vi "Helium Fridge Cool-Down.vi"() -> ()   [LabVIEW 2014]
uses:
  <vilib>/express/express shared/transition.llb/Dynamic To Waveform Array.vi
  <vilib>/express/express signal manip/GetorSetDDTAttributes/Set DDT Attributes/SetT0.vi
  <vilib>/express/express shared/transition.llb/Waveform Array To Dynamic.vi
  <vilib>/express/express signal manip/GetorSetDDTAttributes/Set DDT Attributes/Set DDT Properties.xnode
panel:
  out "Lab Time":string
  out "Most Recent Error":string
  out "Last Sweep Start Time":string
  out "Most Recent Error":string
  out "Last Measurement Taken":string
  out "Run Start Time":string
  in  "Seconds Between\nMeasurements":dbl=30.0
  out "All Clear":bool=TRUE
  out "Error":bool
  out "Heartbeat":bool
  out "?":bool
  in  "stop":bool
  out "Input Triangle Wave":dynamicdata(graph)
  out "Modulator":dynamicdata(graph)
  out "Q Meter":cluster{"Y":dbl[], "Y":dbl[]}[](graph)
  in  "# of Sweeps":dbl=100.0
  out "Resistance Strip Chart":dynamicdata(graph)
  out "Temperature Strip Chart":dynamicdata(graph)
  in  "Heartbeat":bool
  in  "Temp Strip Chart":bool
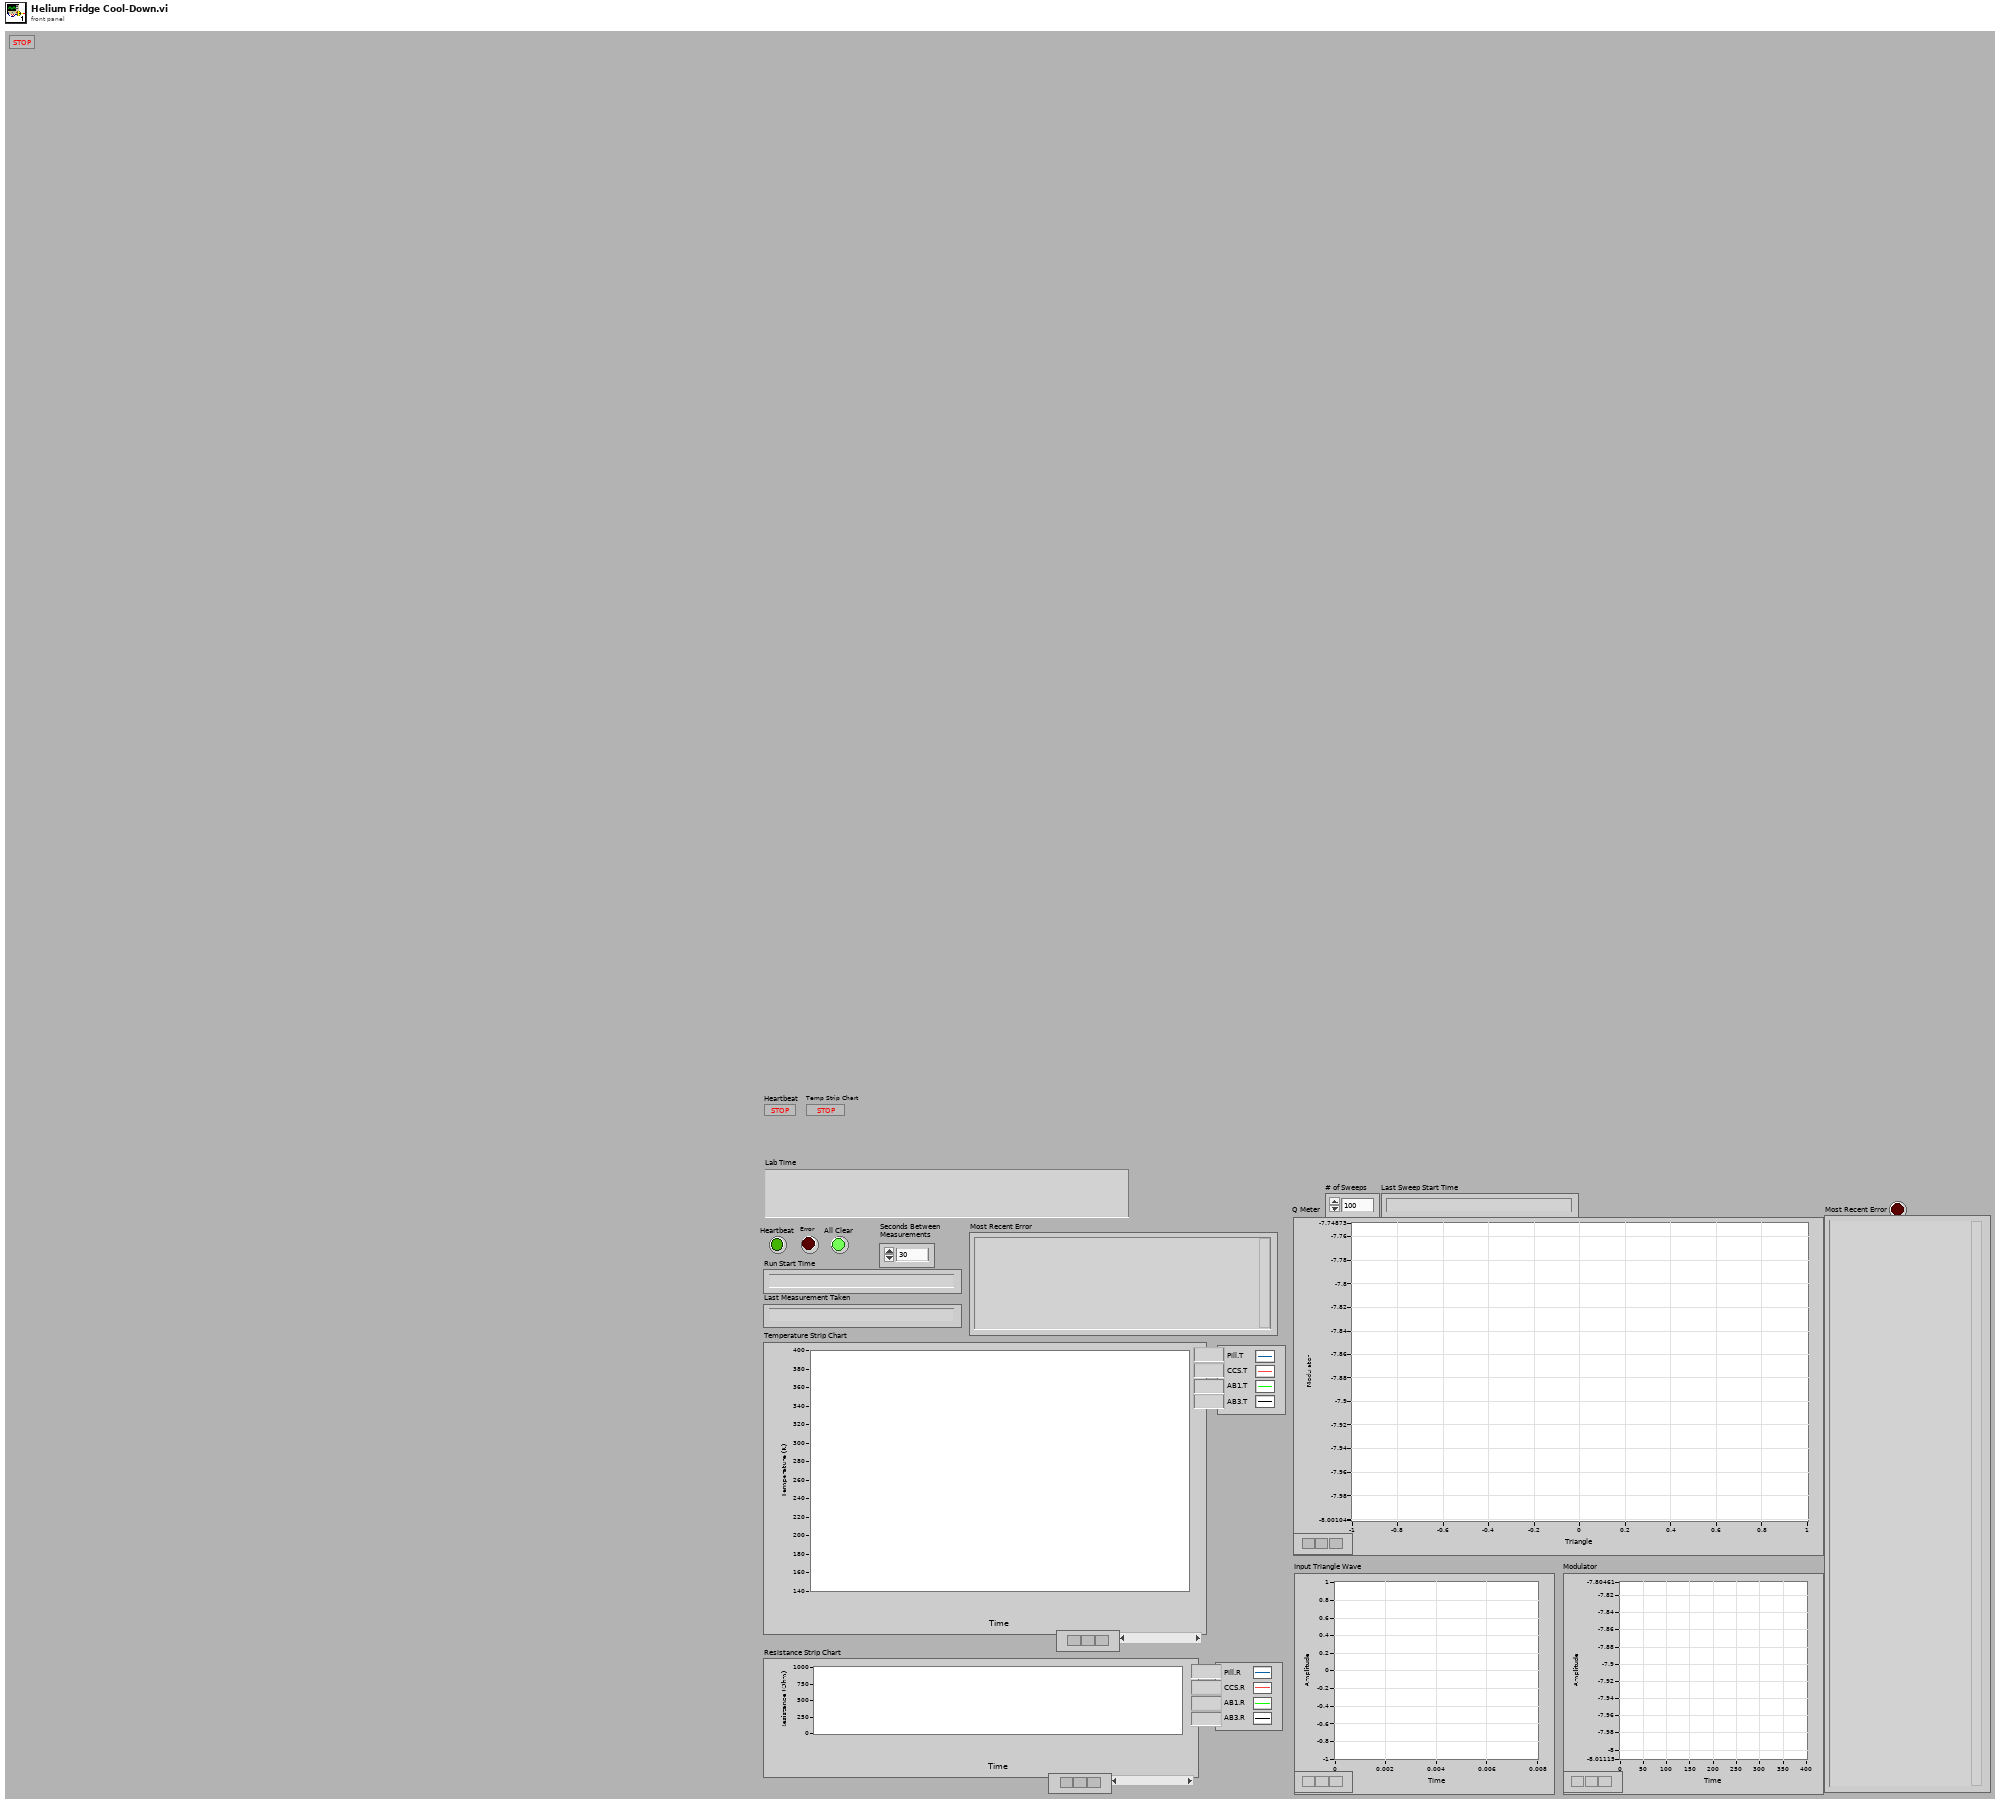
[diagram p1: front panel]
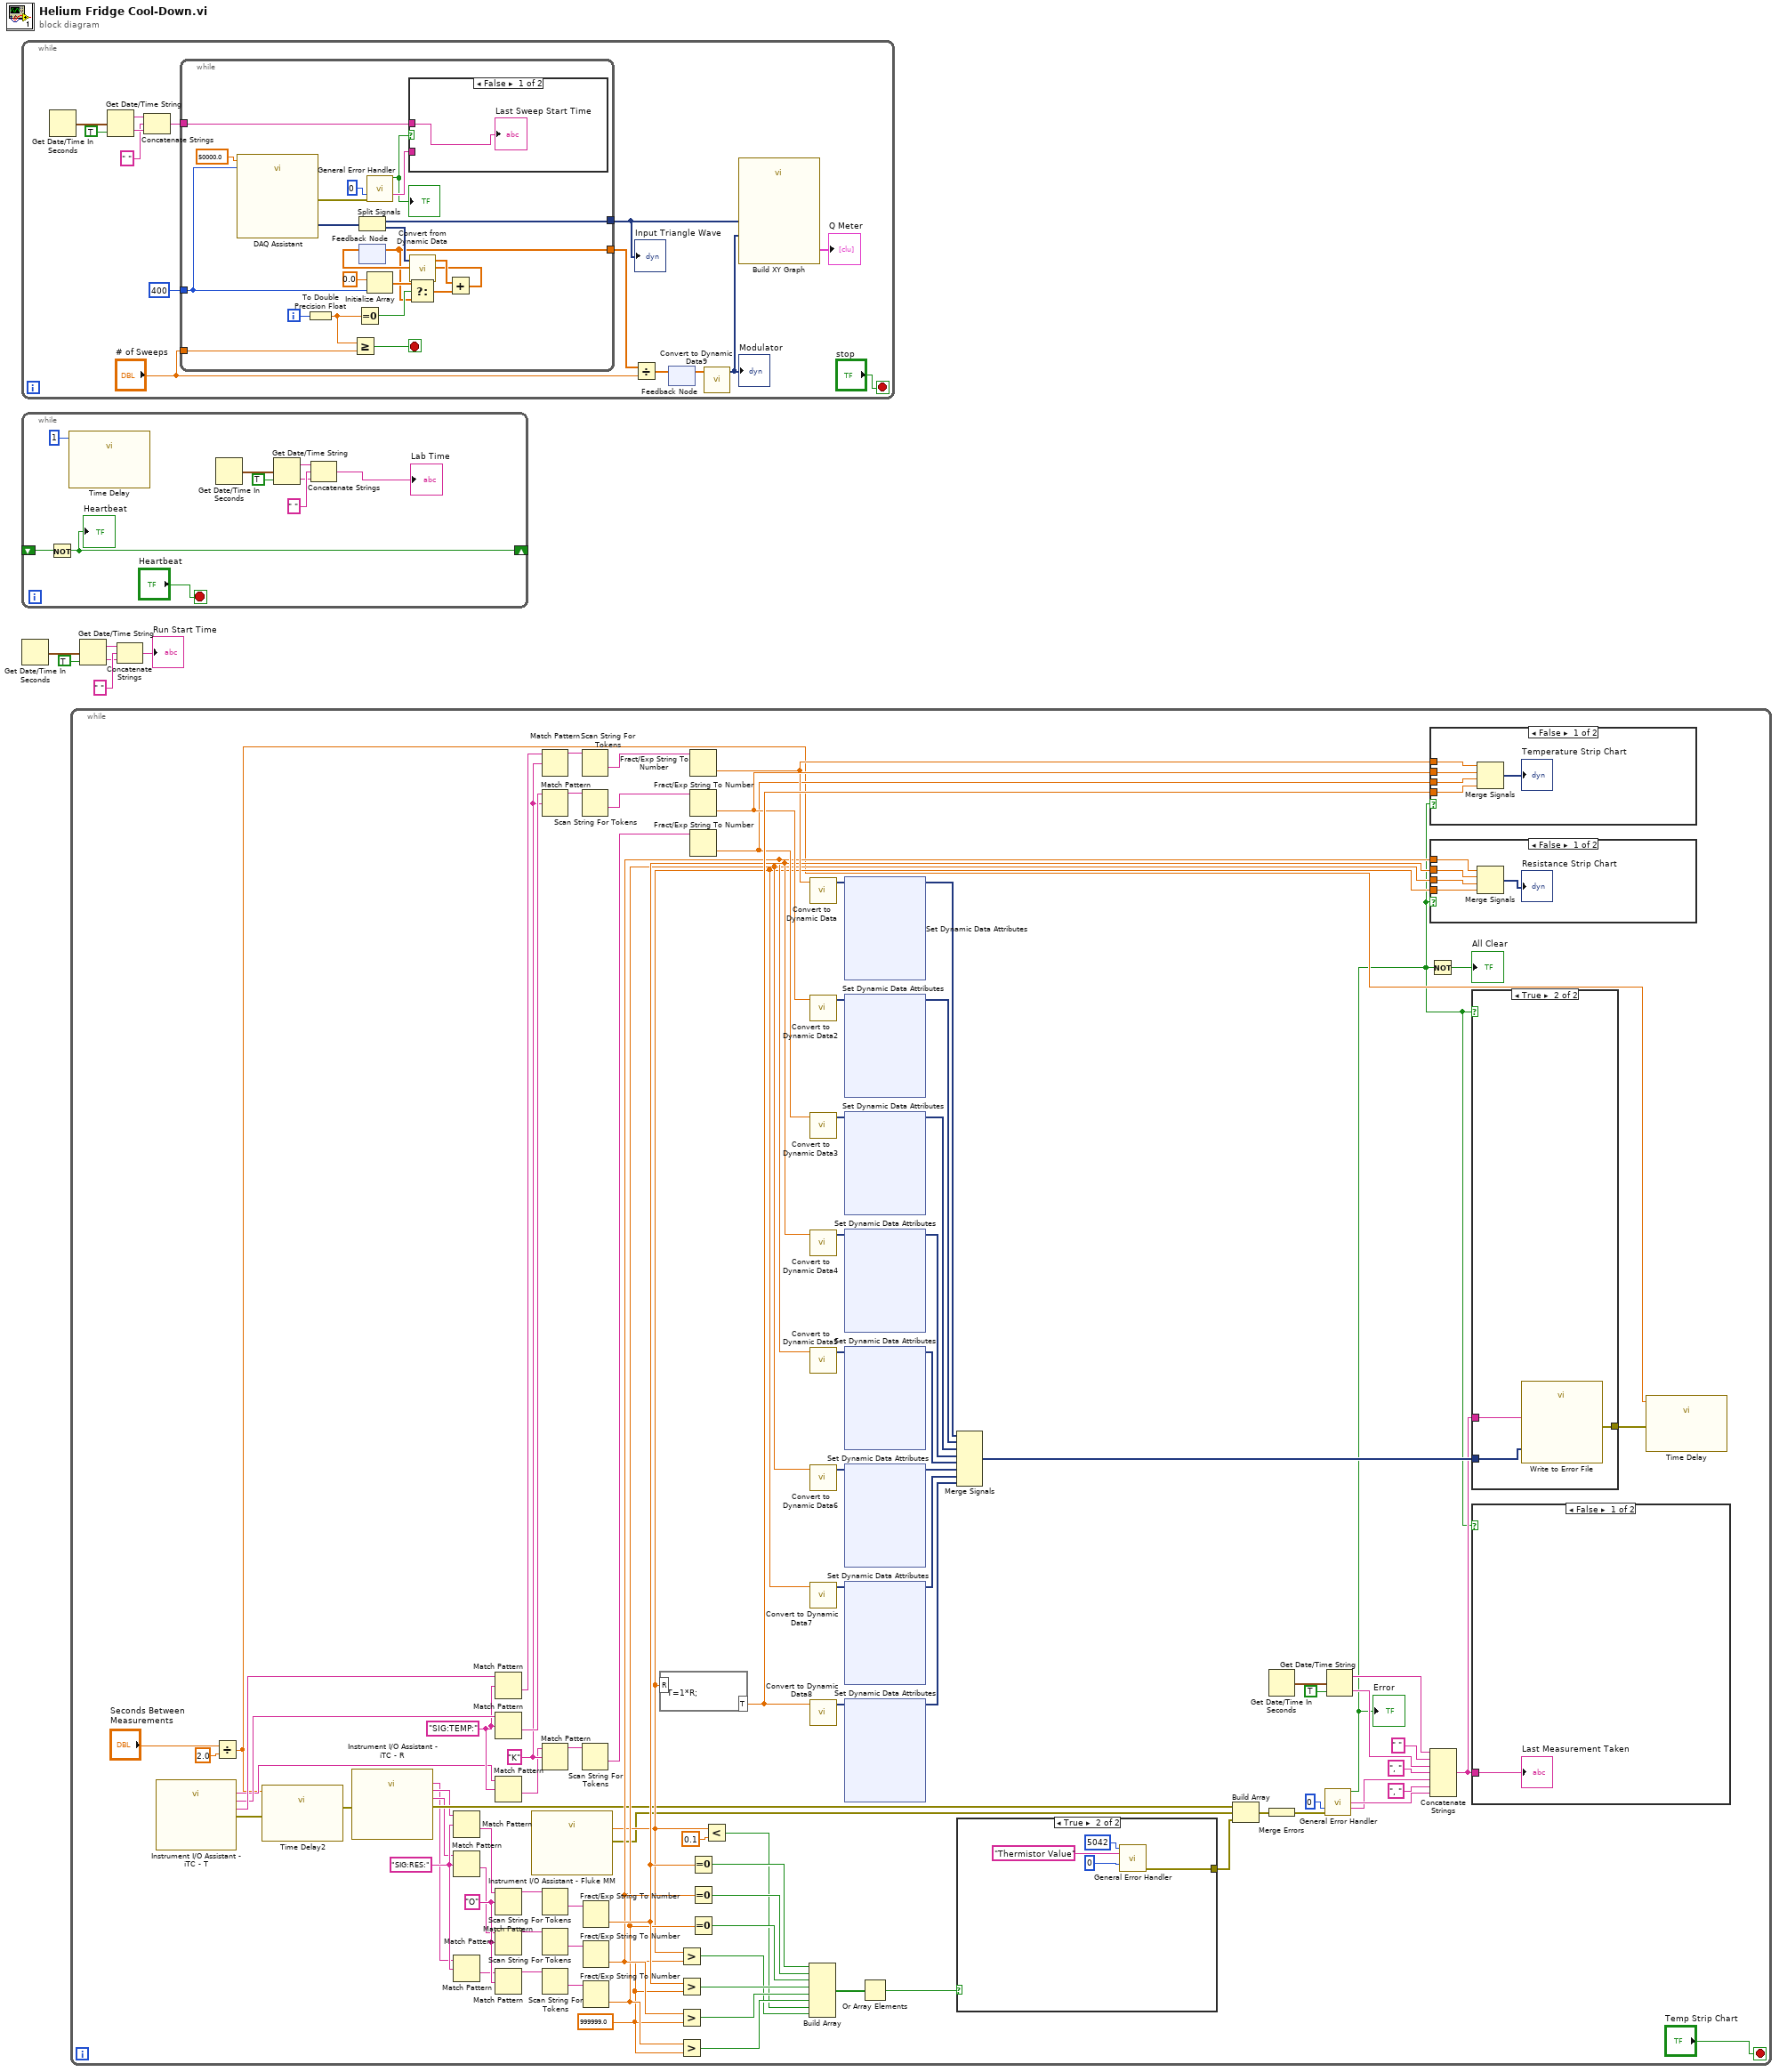
[diagram p0: block diagram]
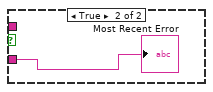
[diagram p2: hidden frame]
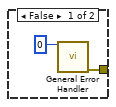
[diagram p3: hidden frame]
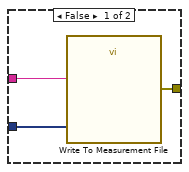
[diagram p6: hidden frame]
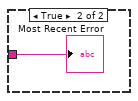
[diagram p7: hidden frame]
diagram:
  n1 = while {
    stop <- "stop" stop-if-true
    n2 = Get Date/Time In Seconds() -> (seconds since 1Jan1904=w8:timestamp)
    n3 = Get Date/Time String(seconds (now)=w8, want seconds? (F)=TRUE) -> (date string=w10:string, time string=w12:string)  [unwired: 1 in]
    n4 = Concatenate Strings(w10, " ", w12) -> (w7:string)
    n5 = while {
      tunnel: "# of Sweeps" -> [w36]
      tunnel: 400 -> [w38]
      tunnel: [w39] -> w13
      tunnel: [w29] -> w18
      tunnel: w7 -> [w22]
      i -> [w37]
      stop <- w28 stop-if-true
      n6 = call "DAQ Assistant"("rate"=50000.0, "number of samples"=w38) -> ("data"=w41:dynamicdata, "error out"=w26:errorcluster)  [unwired: 15 in, 1 out]
      n7 = To Double Precision Float(number=w37) -> (double precision float=w35:dbl)
      n8 = Greater Or Equal?(x=w35, y=w36) -> (x >= y?=w28:bool)
      n9 = Equal To 0?(x=w35) -> (x = 0?=w34:bool)
      n10 = Split Signals(w41) -> (w39:dynamicdata, w40:dynamicdata)  [unwired: 2 in]
      n11 = feedback #1() -> (w29:dbl[])  [unwired: 1 in]
      n12 = call <vilib>:"General Error Handler.vi"("type of dialog (OK msg:1)"=0, "error in (no error)"=w26) -> ("error?"=w24:bool, "message"=w27:string)  [unwired: 9 in, 3 out]
      "?" <- w24
      n13 = Initialize Array(0.0, w38) -> (w32:dbl[])
      n14 = case shown="False" w24 {
        tunnel: w27 -> [_ w44]
        tunnel: w22 -> [w43 _]
        frame False {
          "Last Sweep Start Time" <- w43
        }
        frame True {
          "Most Recent Error" <- w44
        }
      }
      n15 = call "Convert from Dynamic Data"("Dynamic Data Type"=w40) -> ("Array"=w31:dbl[])  [unwired: 3 in]
      n16 = Select(t=w32, s=w34, f=w29) -> (s? t:f=w33:dbl[])
      n17 = Add(x=w31, y=w33) -> (x+y=w30:dbl[])
      n18 = feedback-in #1(w30) -> ()
    }
    "Input Triangle Wave" <- w13
    n19 = Divide(x=w18, y="# of Sweeps") -> (x/y=w16:dbl[])
    n20 = feedback-in #2(w16) -> ()
    n21 = feedback #2() -> (w15:dbl[])  [unwired: 1 in]
    n22 = call "Convert to Dynamic Data9"("Array"=w15) -> ("Dynamic Data Type"=w14:dynamicdata)  [unwired: 3 in]
    "Modulator" <- w14
    n23 = call "Build XY Graph"("Y Input"=w14, "X Input"=w13) -> ("XY Graph"=→"Q Meter":cluster{"Y":dbl[], "Y":dbl[]}[])  [unwired: 8 in, 1 out]
  }
  n24 = while {
    shift-right: [w51] -> _
    shift-left: _ -> [w54]
    stop <- "Heartbeat" stop-if-true
    n25 = Not(x=w54) -> (.not. x?=w51:bool)
    "Heartbeat" <- w51
    n26 = call "Time Delay"("Delay Time (s)"=1) -> ()  [unwired: 10 in, 1 out]
    n27 = Get Date/Time In Seconds() -> (seconds since 1Jan1904=w49:timestamp)
    n28 = Get Date/Time String(seconds (now)=w49, want seconds? (F)=TRUE) -> (date string=w48:string, time string=w46:string)  [unwired: 1 in]
    n29 = Concatenate Strings(w48, " ", w46) -> (→"Lab Time":string)
  }
  n30 = Get Date/Time In Seconds() -> (seconds since 1Jan1904=w5:timestamp)
  n31 = while {
    stop <- "Temp Strip Chart" stop-if-true
    w73 = 999999.0
    w109 = "O"
    w110 = "SIG:RES:"
    w116 = "SIG:TEMP:"
    w115 = "K"
    n32 = call "Instrument I/O Assistant - iTC - T"() -> ("AB1.T"=w114:string, "CCS.T"=w119:string, "Pill.T"=w122:string, "error out"=w63:errorcluster)  [unwired: 23 in, 1 out]
    n33 = Divide(x="Seconds Between\nMeasurements", y=2.0) -> (x/y=w58:dbl)
    n34 = call "Time Delay2"("error in (no error)"=w63, "Delay Time (s)"=w58) -> ("error out"=w64:errorcluster)  [unwired: 9 in]
    n35 = call "Instrument I/O Assistant - iTC - R"("error in"=w64) -> ("AB1.R"=w60:string, "CCS.R"=w61:string, "Pill.R"=w62:string, "error out"=w65:errorcluster)  [unwired: 22 in, 1 out]
    n36 = Match Pattern(string=w61, regular expression=w110) -> (after substring=w108:string)  [unwired: 1 in, 3 out]
    n37 = Match Pattern(string=w62, regular expression=w110) -> (after substring=w107:string)  [unwired: 1 in, 3 out]
    n38 = Match Pattern(string=w60, regular expression=w110) -> (after substring=w106:string)  [unwired: 1 in, 3 out]
    n39 = Match Pattern(string=w122, regular expression=w116) -> (after substring=w121:string)  [unwired: 1 in, 3 out]
    n40 = Match Pattern(string=w119, regular expression=w116) -> (after substring=w118:string)  [unwired: 1 in, 3 out]
    n41 = Match Pattern(string=w114, regular expression=w116) -> (after substring=w113:string)  [unwired: 1 in, 3 out]
    n42 = Match Pattern(string=w108, regular expression=w109) -> (before substring=w105:string)  [unwired: 1 in, 3 out]
    n43 = Match Pattern(string=w107, regular expression=w109) -> (before substring=w104:string)  [unwired: 1 in, 3 out]
    n44 = Match Pattern(string=w106, regular expression=w109) -> (before substring=w103:string)  [unwired: 1 in, 3 out]
    n45 = call "Instrument I/O Assistant - Fluke MM"() -> ("AB3.R"=w71:dbl, "error out"=w68:errorcluster)  [unwired: 25 in, 1 out]
    n46 = Match Pattern(string=w121, regular expression=w115) -> (before substring=w120:string)  [unwired: 1 in, 3 out]
    n47 = Match Pattern(string=w118, regular expression=w115) -> (before substring=w117:string)  [unwired: 1 in, 3 out]
    n48 = Match Pattern(string=w113, regular expression=w115) -> (before substring=w112:string)  [unwired: 1 in, 3 out]
    n49 = Scan String For Tokens(9:w105) -> (1:w102:string)  [unwired: 5 in, 3 out]
    n50 = Scan String For Tokens(9:w104) -> (1:w101:string)  [unwired: 5 in, 3 out]
    n51 = Scan String For Tokens(9:w103) -> (1:w100:string)  [unwired: 5 in, 3 out]
    n52 = Scan String For Tokens(9:w120) -> (1:w144:string)  [unwired: 5 in, 3 out]
    n53 = Scan String For Tokens(9:w117) -> (1:w142:string)  [unwired: 5 in, 3 out]
    n54 = Scan String For Tokens(9:w112) -> (1:w141:string)  [unwired: 5 in, 3 out]
    n55 = Fract/Exp String To Number(string=w102) -> (number=w79:dbl)  [unwired: 3 in, 1 out]
    n56 = Fract/Exp String To Number(string=w101) -> (number=w78:dbl)  [unwired: 3 in, 1 out]
    n57 = Fract/Exp String To Number(string=w100) -> (number=w77:dbl)  [unwired: 3 in, 1 out]
    n58 = formula code="T=1*R;"("R"=w71) -> ("T"=w90:dbl)
    n59 = Greater?(x=w71, y=w73) -> (0:w72:bool)
    n60 = Greater?(x=w79, y=w73) -> (0:w76:bool)
    n61 = Greater?(x=w78, y=w73) -> (0:w75:bool)
    n62 = Greater?(x=w77, y=w73) -> (0:w74:bool)
    n63 = Fract/Exp String To Number(string=w144) -> (number=w81:dbl)  [unwired: 3 in, 1 out]
    n64 = Fract/Exp String To Number(string=w142) -> (number=w82:dbl)  [unwired: 3 in, 1 out]
    n65 = Fract/Exp String To Number(string=w141) -> (number=w80:dbl)  [unwired: 3 in, 1 out]
    n66 = Equal To 0?(x=w79) -> (x = 0?=w87:bool)
    n67 = Equal To 0?(x=w78) -> (x = 0?=w86:bool)
    n68 = Equal To 0?(x=w77) -> (x = 0?=w85:bool)
    n69 = Less?(x=w71, y=0.1) -> (x < y?=w70:bool)
    n70 = Build Array(w87, w86, w85, w76, w75, w74, w70, w72) -> (w84:bool[])
    n71 = call "Convert to Dynamic Data"("Double"=w81) -> ("Dynamic Data Type"=w133:dynamicdata)  [unwired: 3 in]
    n72 = call "Convert to Dynamic Data2"("Double"=w82) -> ("Dynamic Data Type"=w131:dynamicdata)  [unwired: 3 in]
    n73 = call "Convert to Dynamic Data3"("Double"=w80) -> ("Dynamic Data Type"=w130:dynamicdata)  [unwired: 3 in]
    n74 = call "Convert to Dynamic Data4"("Double"=w79) -> ("Dynamic Data Type"=w99:dynamicdata)  [unwired: 3 in]
    n75 = call "Convert to Dynamic Data5"("Double"=w78) -> ("Dynamic Data Type"=w98:dynamicdata)  [unwired: 3 in]
    n76 = call "Convert to Dynamic Data6"("Double"=w77) -> ("Dynamic Data Type"=w97:dynamicdata)  [unwired: 3 in]
    n77 = call "Convert to Dynamic Data7"("Double"=w71) -> ("Dynamic Data Type"=w93:dynamicdata)  [unwired: 3 in]
    n78 = call "Convert to Dynamic Data8"("Double"=w90) -> ("Dynamic Data Type"=w89:dynamicdata)  [unwired: 3 in]
    n79 = xnode "Set Dynamic Data Attributes"("Signals In"=w133) -> ("Signals Out"=w132:dynamicdata)  [unwired: 4 in, 1 out]
    n80 = xnode "Set Dynamic Data Attributes"("Signals In"=w131) -> ("Signals Out"=w129:dynamicdata)  [unwired: 4 in, 1 out]
    n81 = xnode "Set Dynamic Data Attributes"("Signals In"=w130) -> ("Signals Out"=w128:dynamicdata)  [unwired: 4 in, 1 out]
    n82 = xnode "Set Dynamic Data Attributes"("Signals In"=w99) -> ("Signals Out"=w96:dynamicdata)  [unwired: 4 in, 1 out]
    n83 = xnode "Set Dynamic Data Attributes"("Signals In"=w98) -> ("Signals Out"=w95:dynamicdata)  [unwired: 4 in, 1 out]
    n84 = xnode "Set Dynamic Data Attributes"("Signals In"=w97) -> ("Signals Out"=w94:dynamicdata)  [unwired: 4 in, 1 out]
    n85 = xnode "Set Dynamic Data Attributes"("Signals In"=w93) -> ("Signals Out"=w92:dynamicdata)  [unwired: 4 in, 1 out]
    n86 = xnode "Set Dynamic Data Attributes"("Signals In"=w89) -> ("Signals Out"=w88:dynamicdata)  [unwired: 4 in, 1 out]
    n87 = Or Array Elements(Boolean array=w84) -> (logical OR=w83:bool)
    n88 = Merge Signals(w132, w129, w128, w96, w95, w94, w92, w88) -> (w125:dynamicdata)
    n89 = case shown="True" w83 {
      tunnel: [w145 w150] -> w67
      frame False {
        n90 = call <vilib>:"General Error Handler.vi"("[error code] (0)"=0) -> ("error out"=w145:errorcluster)  [unwired: 10 in, 4 out]
      }
      frame True {
        n91 = call <vilib>:"General Error Handler.vi"("[error code] (0)"=5042, "[error source] (\" \")"="Thermistor Value", "type of dialog (OK msg:1)"=0) -> ("error out"=w150:errorcluster)  [unwired: 8 in, 4 out]
      }
    }
    n92 = Build Array(w65, w68, w67) -> (w66:errorcluster[])
    n93 = Get Date/Time In Seconds() -> (seconds since 1Jan1904=w140:timestamp)
    n94 = Merge Errors(w66) -> (w91:errorcluster)
    n95 = call <vilib>:"General Error Handler.vi"("type of dialog (OK msg:1)"=0, "error in (no error)"=w91) -> ("error?"=w57:bool, "source out"=w127:string, "message"=w126:string)  [unwired: 9 in, 2 out]
    "Error" <- w57
    n96 = Get Date/Time String(seconds (now)=w140, want seconds? (F)=TRUE) -> (date string=w138:string, time string=w136:string)  [unwired: 1 in]
    n97 = Not(x=w57) -> (.not. x?=→"All Clear":bool)
    n98 = case shown="False" w57 {
      tunnel: w81 -> [w250 _]
      tunnel: w82 -> [w249 _]
      tunnel: w80 -> [w248 _]
      tunnel: w90 -> [w247 _]
      frame False {
        n99 = Merge Signals(w250, w249, w248, w247) -> (→"Temperature Strip Chart":dynamicdata)
      }
      frame True {
      }
    }
    n100 = case shown="False" w57 {
      tunnel: w78 -> [w245 _]
      tunnel: w79 -> [w244 _]
      tunnel: w77 -> [w243 _]
      tunnel: w71 -> [w242 _]
      frame False {
        n101 = Merge Signals(w245, w244, w243, w242) -> (→"Resistance Strip Chart":dynamicdata)
      }
      frame True {
      }
    }
    n102 = Concatenate Strings(w138, " ", w136, ", ", w126, ", ", w127) -> (w124:string)
    n103 = case shown="True" w57 {
      tunnel: w125 -> [w253 w256]
      tunnel: w124 -> [w252 w255]
      tunnel: [w251 w254] -> w111
      frame False {
        n104 = call "Write To Measurement File"("Signals"=w253, "Comment"=w252) -> ("error out"=w251:errorcluster)  [unwired: 15 in, 2 out]
      }
      frame True {
        n105 = call "Write to Error File"("Signals"=w256, "Comment"=w255) -> ("error out"=w254:errorcluster)  [unwired: 15 in, 2 out]
      }
    }
    n106 = case shown="False" w57 {
      tunnel: w124 -> [w311 w312]
      frame False {
        "Last Measurement Taken" <- w311
      }
      frame True {
        "Most Recent Error" <- w312
      }
    }
    n107 = call "Time Delay"("error in (no error)"=w111, "Delay Time (s)"=w58) -> ()  [unwired: 9 in, 1 out]
  }
  n108 = Get Date/Time String(seconds (now)=w5, want seconds? (F)=TRUE) -> (date string=w4:string, time string=w2:string)  [unwired: 1 in]
  n109 = Concatenate Strings(w4, " ", w2) -> (→"Run Start Time":string)
